vi "3 Logical.vi"() -> ()   [LabVIEW 2015]
panel:
  out "OUT":bool
  in  "STOP":bool
  in  "START":bool
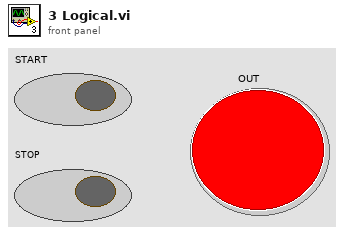
[diagram p1: front panel]
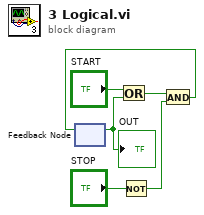
[diagram p0: block diagram]
diagram:
  n1 = feedback #1() -> (w1:bool)  [unwired: 1 in]
  "OUT" <- w1
  n2 = Or(x="START", y=w1) -> (x .or. y?=w4:bool)
  n3 = Not(x="STOP") -> (.not. x?=w3:bool)
  n4 = And(x=w4, y=w3) -> (x .and. y?=w2:bool)
  n5 = feedback-in #1(w2) -> ()
